vi "New Session SetUp.vi"(8 "error in (no error)":errorcluster, 10 "Stop Refnum":refnum<vi>, 11 "Generic Power Analyzer in":refnum<class "Generic Power Analyzer.lvclass">) -> (0 "error out":errorcluster, 3 "Generic Power Analyzer out":refnum<class "Generic Power Analyzer.lvclass">)   [LabVIEW 2014, in "Generic Power Analyzer.lvlib" / "Generic Power Analyzer.lvclass"]
uses:
  Generic Power Analyzer.lvclass
  Subpanel Insertion/Subpanel Inserter.lvclass
panel:
  in  "or":bool
  out "i":i32
  out "Value":bool
  out "ID":string
  in  "Card to Start":u16(ring)
  in  "Voltage":u16(ring)
  in  "Current":u16(ring)
  in  "Wiring":u16(ring)
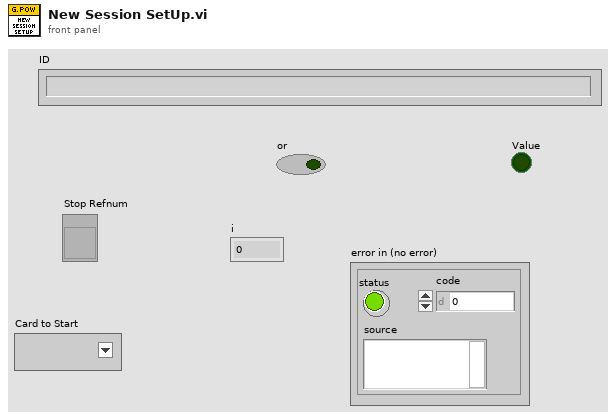
[diagram p1: front panel]
types:
  T1 = typedef "LVStringsAndValuesArrayTypeDef_U16.ctl" = cluster{"String":string, "Value":u16}[]
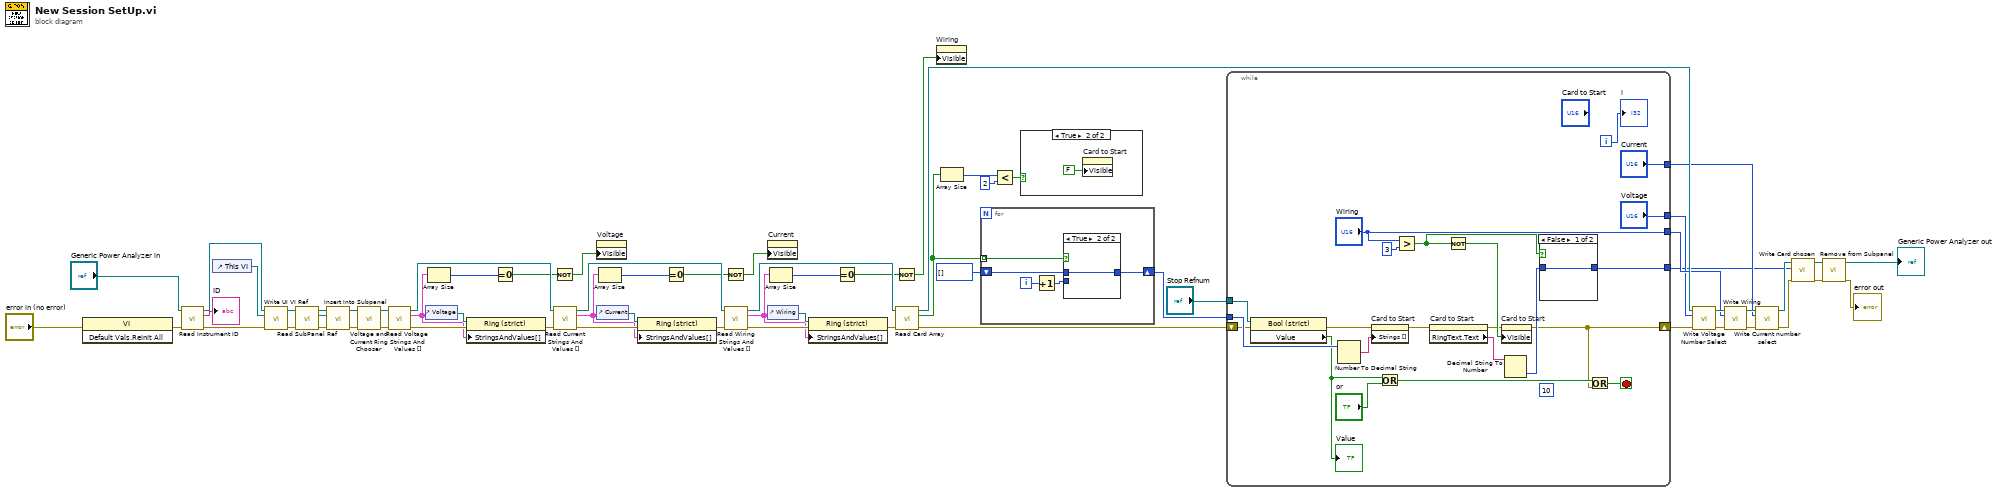
[diagram p0: block diagram]
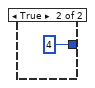
[diagram p3: hidden frame]
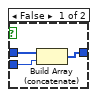
[diagram p4: hidden frame]
diagram:
  n1 = invoke class="VI" method="Default Vals.Reinit All"(error in="error in (no error)") -> (error out=w15:errorcluster)  [unwired: 2 in, 2 out]
  n2 = call-dynamic "Read Instrument ID.vi"("error in (no error)"=w15, "Generic Instrument in"="Generic Power Analyzer in") -> ("error out"=w14:errorcluster, "Instrument ID"=→"ID":string, "Generic Instrument out"=w11:refnum<class "Generic Power Analyzer.lvclass">)  [unwired: 7 in]
  n3 = control-ref of="This VI"() -> (w37:refnum<vi>)
  n4 = call-dynamic "Write UI VI Ref.vi"("error in (no error)"=w14, "UI VI Ref"=w37, "Subpanel Inserter in"=w11) -> ("error out"=w9:errorcluster, "Subpanel Inserter out"=w10:refnum<class "Generic Power Analyzer.lvclass">)  [unwired: 7 in]
  n5 = call-dynamic "Read SubPanel Ref.vi"("error in (no error)"=w9, "Subpanel Inserter in"=w10) -> ("error out"=w6:errorcluster, "SubPanel Ref"=w7:refnum<vi>, "Subpanel Inserter out"=w8:refnum<class "Generic Power Analyzer.lvclass">)  [unwired: 7 in]
  n6 = call "Insert Into Subpanel.vi"("Error In"=w6, "SubPanel Ref"=w7, "Subpanel Inserter"=w8) -> ("error out"=w31:errorcluster, "Subpanel Inserter"=w29:refnum<class "Generic Power Analyzer.lvclass">)  [unwired: 7 in]
  n7 = call-dynamic "Voltage and Current Ring Chooser.vi"("error in (no error)"=w31, "Generic Power Analyzer in"=w29) -> ("error out"=w30:errorcluster, "Generic Power Analyzer out"=w28:refnum<class "Generic Power Analyzer.lvclass">)  [unwired: 8 in]
  n8 = call-dynamic "Read Voltage Strings And Values [].vi"("error in (no error)"=w30, "Generic Power Analyzer in"=w28) -> ("error out"=w45:errorcluster, "Strings And Values []"=w27:T1, "Generic Power Analyzer out"=w59:refnum<class "Generic Power Analyzer.lvclass">)  [unwired: 7 in]
  n9 = control-ref of="Voltage"() -> (w62:refnum<vi>)
  n10 = Array Size(array=w27) -> (size(s)=w26:i32)
  n11 = property class="Ring (strict)"(reference=w62, error in=w45, "StringsAndValues[]"=w27) -> (error out=w44:errorcluster)  [unwired: 1 out]
  n12 = Equal To 0?(x=w26) -> (x = 0?=w25:bool)
  n13 = Not(x=w25) -> (.not. x?=w24:bool)
  n14 = call-dynamic "Read Current Strings And Values [].vi"("error in (no error)"=w44, "Generic Power Analyzer in"=w59) -> ("error out"=w43:errorcluster, "Strings And Values []"=w19:T1, "Generic Power Analyzer out"=w58:refnum<class "Generic Power Analyzer.lvclass">)  [unwired: 7 in]
  n15 = property on="Voltage" class="Ring (strict)"("Visible"=w24) -> ()  [unwired: 2 in, 2 out]
  n16 = control-ref of="Current"() -> (w61:refnum<vi>)
  n17 = Array Size(array=w19) -> (size(s)=w23:i32)
  n18 = property class="Ring (strict)"(reference=w61, error in=w43, "StringsAndValues[]"=w19) -> (error out=w42:errorcluster)  [unwired: 1 out]
  n19 = Equal To 0?(x=w23) -> (x = 0?=w22:bool)
  n20 = Not(x=w22) -> (.not. x?=w18:bool)
  n21 = call-dynamic "Read Wiring Strings And Values [].vi"("error in (no error)"=w42, "Generic Power Analyzer in"=w58) -> ("error out"=w41:errorcluster, "Strings And Values []"=w17:T1, "Generic Power Analyzer out"=w57:refnum<class "Generic Power Analyzer.lvclass">)  [unwired: 7 in]
  n22 = property on="Current" class="Ring (strict)"("Visible"=w18) -> ()  [unwired: 2 in, 2 out]
  n23 = control-ref of="Wiring"() -> (w60:refnum<vi>)
  n24 = Array Size(array=w17) -> (size(s)=w21:i32)
  n25 = property class="Ring (strict)"(reference=w60, error in=w41, "StringsAndValues[]"=w17) -> (error out=w40:errorcluster)  [unwired: 1 out]
  n26 = Equal To 0?(x=w21) -> (x = 0?=w20:bool)
  n27 = Not(x=w20) -> (.not. x?=w16:bool)
  n28 = call-dynamic "Read Card Array.vi"("error in (no error)"=w40, "Generic Instrument in"=w57) -> ("error out"=w39:errorcluster, "Card Array"=w35:bool[], "Generic Instrument out"=w53:refnum<class "Generic Power Analyzer.lvclass">)  [unwired: 7 in]
  n29 = property on="Wiring" class="Ring (strict)"("Visible"=w16) -> ()  [unwired: 2 in, 2 out]
  n30 = Array Size(array=w35) -> (size(s)=w34:i32)
  n31 = for {
    tunnel: w35 -> [w69] mode=indexing
    shift-right: [w65] -> w63
    shift-left: i32[] [] -> [w68]
    i -> [w67]
    n32 = Increment(x=w67) -> (x+1=w66:i32)
    n33 = case shown="True" w69 {
      tunnel: w68 -> [w72 w73]
      tunnel: w66 -> [w71 _]
      tunnel: [w70 w73] -> w65
      frame False {
        n34 = Build Array (concatenate)(w72, w71) -> (w70:i32[])
      }
      frame True {
      }
    }
  }
  n35 = Less?(x=w34, y=2) -> (x < y?=w32:bool)
  n36 = case shown="True" w32 {
    frame False {
    }
    frame True {
      n37 = property on="Card to Start" class="Ring (strict)"("Visible"=FALSE) -> ()  [unwired: 2 in, 2 out]
    }
  }
  n38 = while {
    tunnel: w63 -> [w96]
    tunnel: ["Wiring"] -> w49
    tunnel: ["Voltage"] -> w48
    tunnel: ["Current"] -> w47
    tunnel: [w86] -> w46
    shift-right: [w79] -> w38
    shift-left: w39 -> [w77]
    tunnel: "Stop Refnum" -> [w75]
    i -> [w83]
    stop <- w78 stop-if-true
    (unwired) 10
    n39 = property class="Bool (strict)"(reference=w75, error in=w77) -> (error out=w76:errorcluster, "Value"=w82:bool)  [unwired: 1 out]
    "Value" <- w82
    n40 = Number To Decimal String(number=w96) -> (decimal integer string=w95:string[])  [unwired: 1 in]
    n41 = property on="Card to Start" class="Ring (strict)"(error in=w76, "Strings []"=w95) -> (error out=w85:errorcluster)  [unwired: 1 in, 1 out]
    n42 = Or(x=w82, y="or") -> (x .or. y?=w80:bool)
    n43 = Greater?(x="Wiring", y=u16 3) -> (0:w91:bool)
    n44 = property on="Card to Start" class="Ring (strict)"(error in=w85) -> (error out=w84:errorcluster, "RingText.Text"=w94:string)  [unwired: 1 in, 1 out]
    n45 = Not(x=w91) -> (.not. x?=w92:bool)
    n46 = property on="Card to Start" class="Ring (strict)"(error in=w84, "Visible"=w92) -> (error out=w79:errorcluster)  [unwired: 1 in, 1 out]
    n47 = Decimal String To Number(string=w94) -> (number=w90:i32)  [unwired: 2 in, 1 out]
    n48 = case shown="False" w91 {
      tunnel: w90 -> [w97 _]
      tunnel: [w97 4] -> w86
      frame False {
      }
      frame True {
      }
    }
    n49 = Or(x=w80, y=w79) -> (x .or. y?=w78:bool)
    "i" <- w83
  }
  n50 = call-dynamic "Write Voltage Number Select.vi"("error in (no error)"=w38, "Voltage Number Select"=w48, "Generic Power Analyzer in"=w53) -> ("error out"=w56:errorcluster, "Generic Power Analyzer out"=w52:refnum<class "Generic Power Analyzer.lvclass">)  [unwired: 7 in]
  n51 = call-dynamic "Write Wiring .vi"("error in (no error)"=w56, "Wiring"=w49, "Generic Power Analyzer in"=w52) -> ("error out"=w55:errorcluster, "Generic Power Analyzer out"=w51:refnum<class "Generic Power Analyzer.lvclass">)  [unwired: 7 in]
  n52 = call-dynamic "Write Current number select.vi"("error in (no error)"=w55, "Current number select"=w47, "Generic Power Analyzer in"=w51) -> ("error out"=w54:errorcluster, "Generic Power Analyzer out"=w50:refnum<class "Generic Power Analyzer.lvclass">)  [unwired: 7 in]
  n53 = call-dynamic "Write Card chosen.vi"("error in (no error)"=w54, "Card chosen"=w46, "Generic Power Analyzer in"=w50) -> ("error out"=w3:errorcluster, "Generic Power Analyzer out"=w4:refnum<class "Generic Power Analyzer.lvclass">)  [unwired: 7 in]
  n54 = call-dynamic "Remove from Subpanel.vi"("Error In"=w3, "Subpanel Inserter"=w4) -> ("error out"=→"error out":errorcluster, "Subpanel Inserter 2"=→"Generic Power Analyzer out":refnum<class "Generic Power Analyzer.lvclass">)  [unwired: 8 in]
